vi "Write Current Command Code.vi"(8 "error in (no error)":errorcluster, 10 "Current Command Code":string, 11 "AK TCP in":refnum<class "AK TCP.lvclass">) -> (0 "error out":errorcluster, 3 "AK TCP out":refnum<class "AK TCP.lvclass">)   [LabVIEW 2023, in "Protocols.lvlib" / "AK TCP.lvclass"]
uses:
  AK TCP.lvclass
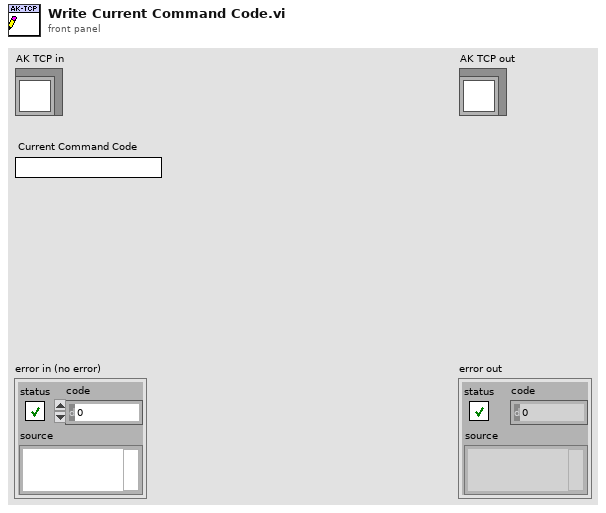
[diagram p1: front panel]
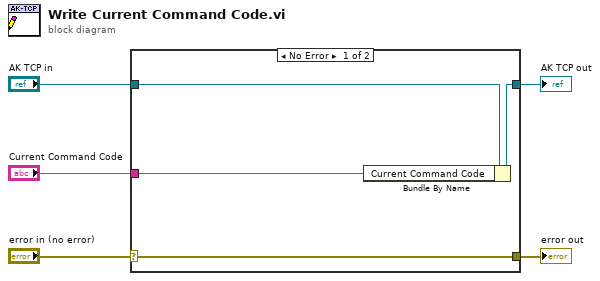
[diagram p0: block diagram]
diagram:
  n1 = case shown="No Error" "error in (no error)" {
    selector: "error in (no error)" -> [w9 w10]
    tunnel: [w9 w10] -> w4
    tunnel: [w7 w11] -> w2
    tunnel: "AK TCP in" -> [w8 w11]
    tunnel: "Current Command Code" -> [w6 _]
    frame No Error {
      n2 = Bundle By Name(cluster=w8, "Current Command Code"=w6) -> (w7:refnum<class "AK TCP.lvclass">)
    }
    frame Error {
    }
  }
  "error out" <- w4
  "AK TCP out" <- w2
